vi "Update Client Data Representation.vi"(8 "error in (no error)":errorcluster, 11 "Control-Client in":refnum<class "Control-Client.lvclass">) -> (0 "error out":errorcluster, 3 "Control-Client out":refnum<class "Control-Client.lvclass">)   [LabVIEW 2019, in "Control-Client.lvclass"]
uses:
  Control-Client.lvclass
  Control-Client.lvclass/Control-Client.ctl
  methods/Read Group #.vi
  Experiments/Experiments_group.lvclass
  Experiments/Experiment.lvclass
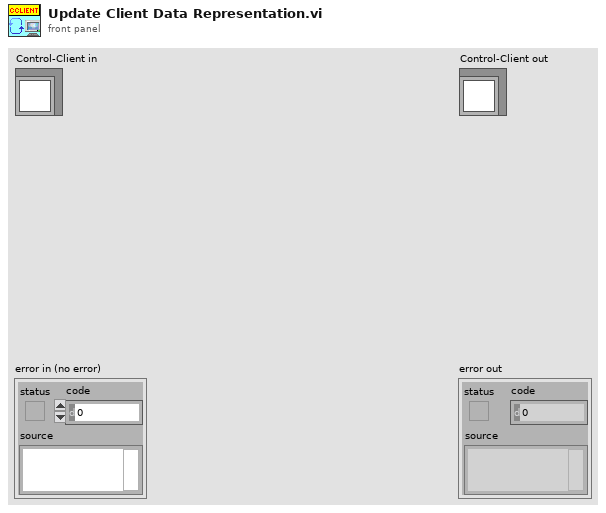
[diagram p1: front panel]
types:
  T1 = typedef "Control-Client.lvclass/Delays-refs_CLIENT.ctl" = cluster{"# points":refnum<vi>, "Step, ps":refnum<vi>, "OZ, ps":refnum<vi>, "# current":refnum<vi>, "RDT, ps":refnum<vi>, "Total length, ps":refnum<vi>, "Kinetics length, ps":refnum<vi>, "Real zero, ps":refnum<vi>, "# par point":refnum<vi>}
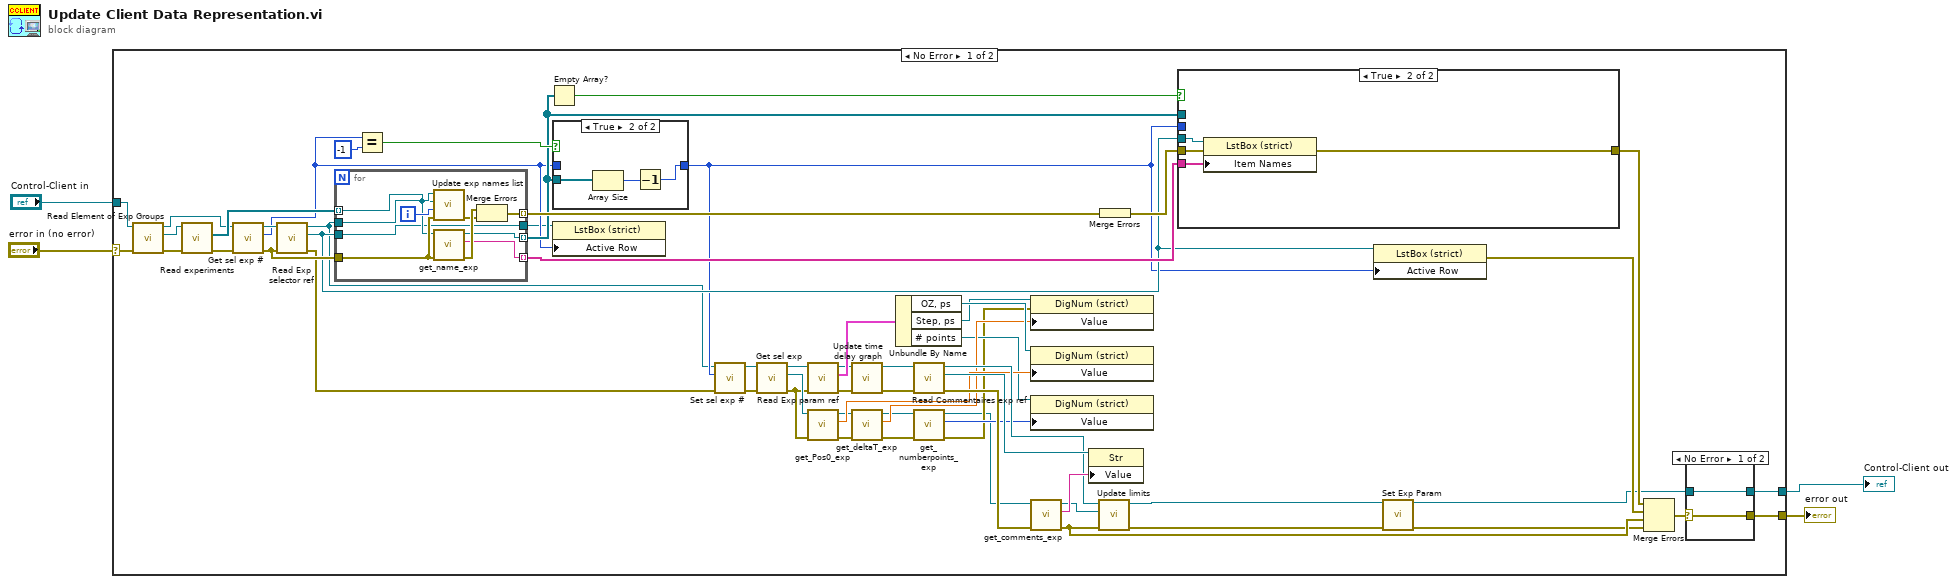
[diagram p0: block diagram]
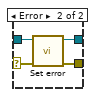
[diagram p2: hidden frame]
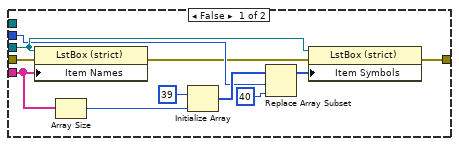
[diagram p4: hidden frame]
diagram:
  n1 = case shown="No Error" "error in (no error)" {
    selector: "error in (no error)" -> [w62 w100]
    tunnel: [w6 w100] -> w3
    tunnel: [w7 w99] -> w1
    tunnel: "Control-Client in" -> [w63 w99]
    frame No Error {
      n2 = call "Read Element of Exp Groups.vi"("error in (no error)"=w62, "Control-Client in"=w63) -> ("error out"=w60:errorcluster, "Experiments_group.lvclass"=w61:refnum<class "Experiments_group.lvclass">, "Control-Client out"=w56:refnum<class "Control-Client.lvclass">)  [unwired: 7 in]
      n3 = call "Read experiments.vi"("error in (no error)"=w60, "Experiments_group.lvclass in"=w61) -> ("error out"=w58:errorcluster, "Experiments"=w59:refnum<class "Experiment.lvclass">[])  [unwired: 6 in, 1 out]
      n4 = call "Get sel exp #.vi"("error in (no error)"=w58, "Control-Client in"=w56) -> ("error out"=w57:errorcluster, "Exp sel #"=w38:i32, "Control-Client out"=w55:refnum<class "Control-Client.lvclass">)  [unwired: 7 in]
      n5 = call "Read Exp selector ref.vi"("error in (no error)"=w57, "Control-Client in"=w55) -> ("error out"=w35:errorcluster, "Exp selector ref"=w39:refnum<vi>, "Control-Client out"=w5:refnum<class "Control-Client.lvclass">)  [unwired: 7 in]
      n6 = for {
        tunnel: w39 -> [w74]
        tunnel: w59 -> [w75] mode=indexing
        tunnel: w5 -> [w83]
        tunnel: w57 -> [w77]
        tunnel: [w80] -> w50 mode=indexing
        tunnel: [w79] -> w46 mode=indexing
        tunnel: [w78] -> w40 mode=indexing
        tunnel: [w74] -> w37
        i -> [w76]
        n7 = call "Update exp names list.vi"("error in (no error)"=w77, "# row"=w76, "Experiment in"=w75, "Control-Client in"=w83) -> ("error out"=w81:errorcluster)  [unwired: 6 in, 1 out]
        n8 = call "get_name_exp.vi"("error in (no error)"=w77, "Experiment.lvclass in"=w75) -> ("error out"=w82:errorcluster, "Exp name"=w78:string, "Experiment.lvclass out"=w79:refnum<class "Experiment.lvclass">)  [unwired: 7 in]
        n9 = Merge Errors(w82, w81) -> (w80:errorcluster)
      }
      n10 = Equal?(x=w38, y=-1) -> (x = y?=w47:bool)
      n11 = Empty Array?(array=w46) -> (empty?=w54:bool)
      n12 = case shown="True" w47 {
        tunnel: [w70 w71] -> w36
        tunnel: w38 -> [w70 _]
        tunnel: w46 -> [_ w73]
        frame False {
        }
        frame True {
          n13 = Array Size(array=w73) -> (size(s)=w72:i32)
          n14 = Decrement(x=w72) -> (x-1=w71:i32)
        }
      }
      n15 = property class="LstBox (strict)"(reference=w37, "Active Row"=w38) -> ()  [unwired: 1 in, 2 out]
      n16 = call "Set sel exp #.vi"("error in (no error)"=w35, "Exp sel #"=w36, "Control-Client in"=w5) -> ("error out"=w24:errorcluster, "Control-Client out"=w22:refnum<class "Control-Client.lvclass">)  [unwired: 7 in]
      n17 = call "Get sel exp.vi"("error in (no error)"=w24, "Control-Client in"=w22) -> ("error out"=w16:errorcluster, "Sel experiment"=w23:refnum<class "Experiment.lvclass">, "Control-Client out"=w21:refnum<class "Control-Client.lvclass">)  [unwired: 7 in]
      n18 = call "Read Exp param ref.vi"("error in (no error)"=w16, "Control-Client in"=w21) -> ("error out"=w20:errorcluster, "Exp param ref"=w32:T1, "Control-Client out"=w19:refnum<class "Control-Client.lvclass">)  [unwired: 7 in]
      n19 = call "get_Pos0_exp.vi"("error in (no error)"=w16, "Experiment.lvclass in"=w23) -> ("error out"=w14:errorcluster, "Delay0,ps"=w30:dbl, "Experiment.lvclass out"=w15:refnum<class "Experiment.lvclass">)  [unwired: 6 in]
      n20 = call "Update time delay graph.vi"("error in (no error)"=w20, "Control-Client en entrée"=w19) -> ("error out"=w18:errorcluster, "Control-Client en sortie"=w17:refnum<class "Control-Client.lvclass">)  [unwired: 8 in]
      n21 = call "get_deltaT_exp.vi"("error in (no error)"=w14, "Experiment.lvclass in"=w15) -> ("error out"=w13:errorcluster, "deltaTlast"=w28:dbl, "Experiment.lvclass out"=w12:refnum<class "Experiment.lvclass">)  [unwired: 7 in]
      n22 = Unbundle By Name(w32) -> ("OZ, ps"=w31:refnum<vi>, "Step, ps"=w29:refnum<vi>, "# points"=w27:refnum<vi>)
      n23 = call "Read Commentaires exp ref.vi"("error in (no error)"=w18, "Control-Client in"=w17) -> ("error out"=w51:errorcluster, "Commentaires exp ref"=w52:refnum<vi>, "Control-Client out"=w41:refnum<class "Control-Client.lvclass">)  [unwired: 7 in]
      n24 = call "get_numberpoints_exp.vi"("error in (no error)"=w13, "Experiment.lvclass in"=w12) -> ("error out"=w25:errorcluster, "numberpoints"=w26:i32, "Experiment.lvclass out"=w11:refnum<class "Experiment.lvclass">)  [unwired: 7 in]
      n25 = property class="DigNum (strict)"(reference=w29, error in=w25, "Value"=w28) -> ()  [unwired: 2 out]
      n26 = property class="DigNum (strict)"(reference=w31, "Value"=w30) -> ()  [unwired: 1 in, 2 out]
      n27 = property class="DigNum (strict)"(reference=w27, "Value"=w26) -> ()  [unwired: 1 in, 2 out]
      n28 = call "get_comments_exp.vi"("error in (no error)"=w51, "Experiment.lvclass in"=w11) -> ("error out"=w42:errorcluster, "Comments"=w53:string, "Experiment.lvclass out"=w43:refnum<class "Experiment.lvclass">)  [unwired: 7 in]
      n29 = property class="Str"(reference=w52, "Value"=w53) -> ()  [unwired: 1 in, 2 out]
      n30 = call "Update limits.vi"("error in (no error)"=w42, "Experiment.lvclass in"=w43, "Control-Client in"=w41) -> ("error out"=w33:errorcluster, "Control-Client out"=w34:refnum<class "Control-Client.lvclass">)  [unwired: 7 in]
      n31 = Merge Errors(w50) -> (w49:errorcluster)
      n32 = case shown="True" w54 {
        tunnel: w46 -> [_ _]
        tunnel: w39 -> [w89 w98]
        tunnel: w36 -> [w88 _]
        tunnel: w49 -> [w87 w97]
        tunnel: [w85 w96] -> w45
        tunnel: w40 -> [w84 w95]
        frame False {
          n33 = property on="Property Node" class="LstBox (strict)"(reference=w89, error in=w87, "Item Names"=w84) -> (error out=w86:errorcluster)  [unwired: 1 out]
          n34 = Array Size(array=w84) -> (size(s)=w90:i32)
          n35 = Initialize Array(39, w90) -> (w92:i32[])
          n36 = Replace Array Subset(array=w92, new element=40 ("new element/subarray"), index=w88) -> (w91:i32[])
          n37 = property on="Property Node" class="LstBox (strict)"(reference=w89, error in=w86, "Item Symbols"=w91) -> (error out=w85:errorcluster)  [unwired: 1 out]
        }
        frame True {
          n38 = property on="Property Node" class="LstBox (strict)"(reference=w98, error in=w97, "Item Names"=w95) -> (error out=w96:errorcluster)  [unwired: 1 out]
        }
      }
      n39 = property on="Property Node" class="LstBox (strict)"(reference=w39, "Active Row"=w36) -> (error out=w44:errorcluster)  [unwired: 1 in, 1 out]
      n40 = call "Set Exp Param.vi"("Control-Client in"=w34, "error in (no error)"=w33) -> ("Control-Client out"=w9:refnum<class "Control-Client.lvclass">, "error out"=w10:errorcluster)  [unwired: 12 in]
      n41 = Merge Errors(w45, w44, w42, w10) -> (w8:errorcluster)
      n42 = case shown="No Error" w8 {
        selector: w8 -> [w65 w66]
        tunnel: w9 -> [w64 w69]
        tunnel: [w65 w68] -> w6
        tunnel: [w64 w67] -> w7
        frame No Error {
        }
        frame Error {
          n43 = call "Set error.vi"("error in (no error)"=w66, "Control-Client in"=w69) -> ("error out"=w68:errorcluster, "Control-Client out"=w67:refnum<class "Control-Client.lvclass">)  [unwired: 8 in]
        }
      }
    }
    frame Error {
    }
  }
  "error out" <- w3
  "Control-Client out" <- w1
